vi "LookForStartOfMessage.vi"(8 "error in (no error)":errorcluster, 11 "TCP_Client in":refnum<class "TCP_Client.lvclass">) -> (0 "error out":errorcluster, 3 "TCP_Client out":refnum<class "TCP_Client.lvclass">)   [LabVIEW 2023, in "TCP_Client.lvlib" / "TCP_Client.lvclass"]
uses:
  TCP_Client.lvclass
  C:/Program Files (x86)/National Instruments/LabVIEW 2023/vi.lib/ActorFramework/Actor/Actor.lvclass
  <vilib>/ActorFramework/Actor/Actor.lvclass/Actor.ctl
  <vilib>/ActorFramework/Message Enqueuer/Message Enqueuer.lvclass/Message Enqueuer.ctl
  TCP_Client.lvclass/TCP_Client.ctl
  TCP_Client Messages/DisabelConnectButton Msg/DisabelConnectButton Msg.lvclass/DisabelConnectButton Msg.ctl
  <vilib>/ActorFramework/Message Enqueuer/Init from Existing Queue.vi
  <vilib>/ActorFramework/Message Enqueuer/Enqueue.vi
  TCP_Client Messages/LookForStartOfMessage Msg/LookForStartOfMessage Msg.lvclass
  C:/Program Files (x86)/National Instruments/LabVIEW 2023/vi.lib/ActorFramework/Message/Message.lvclass
  TCP_Client Messages/GetMessageLength Msg/GetMessageLength Msg.lvclass
  TCP_Client Messages/DisabelConnectButton Msg/DisabelConnectButton Msg.lvclass
  <vilib>/ActorFramework/Message Priority Queue/Priority Enqueue.vi
  <vilib>/ActorFramework/Message Enqueuer/Message Enqueuer.lvclass
  <vilib>/ActorFramework/Actor/Actor.lvclass
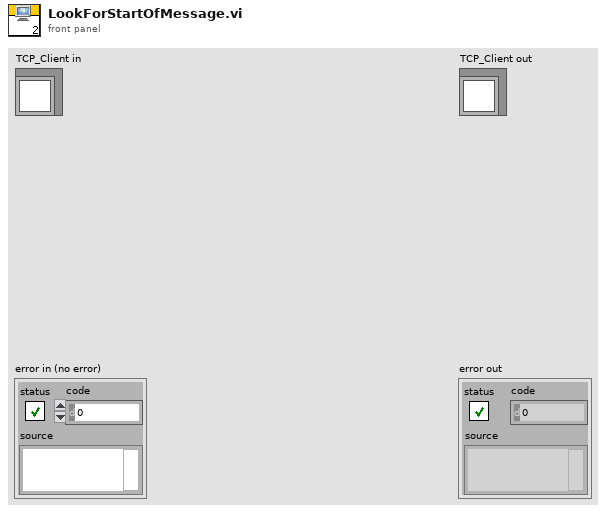
[diagram p1: front panel]
types:
  T1 = enum8{"Enabled", "Disabled", "Disabled and Grayed Out"}
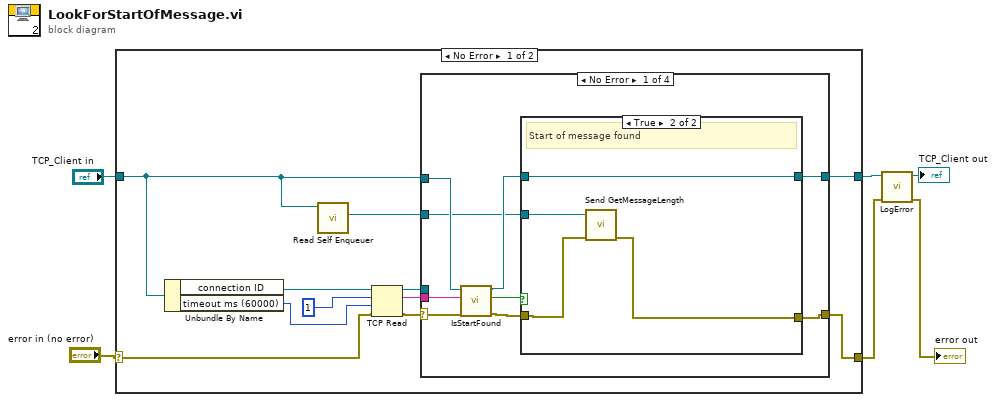
[diagram p0: block diagram]
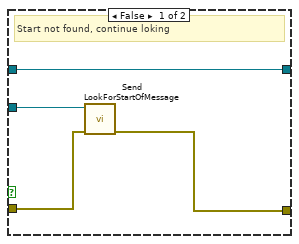
[diagram p2: hidden frame]
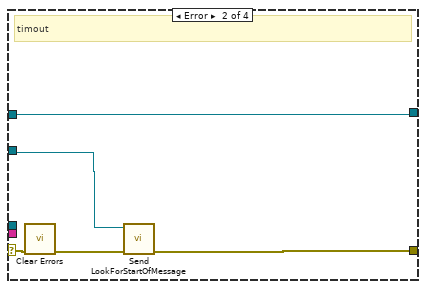
[diagram p3: hidden frame]
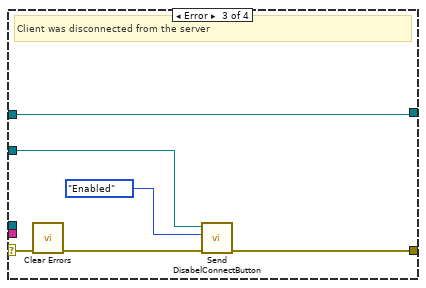
[diagram p4: hidden frame]
diagram:
  n1 = case shown="No Error" "error in (no error)" {
    selector: "error in (no error)" -> [w14 w49]
    tunnel: [w11 w49] -> w2
    tunnel: [w8 w48] -> w4
    tunnel: "TCP_Client in" -> [w9 w48]
    frame No Error {
      n2 = Unbundle By Name(w9) -> ("connection ID"=w17:refnum<k5>, "timeout ms (60000)"=w15:i32)
      n3 = call <vilib>:"Read Self Enqueuer.vi"("Actor"=w9) -> ("Self Enqueuer"=w10:refnum<class "Message Enqueuer.lvclass">)  [unwired: 10 in]
      n4 = TCP Read(connection ID=w17, bytes to read=1, error in (no error)=w14, 9:w15) -> (connection ID out=w13:refnum<k5>, data out=w12:string, error out=w7:errorcluster)  [unwired: 1 in]
      n5 = case shown="No Error" w7 {
        selector: w7 -> [w24 w39 w41 w46]
        tunnel: w13 -> [_ _ _ _]
        tunnel: w12 -> [w25 _ _ _]
        tunnel: [w20 w36 w42 w46] -> w11
        tunnel: w10 -> [w18 w35 w44 _]
        tunnel: w9 -> [w26 w38 w45 w47]
        tunnel: [w19 w38 w45 w47] -> w8
        frame No Error {
          n6 = call "IsStartFound.vi"("error in (no error)"=w24, "data in"=w25, "TCP_Client in"=w26) -> ("error out"=w21:errorcluster, "StartOfMessage"=w23:bool, "TCP_Client out"=w22:refnum<class "TCP_Client.lvclass">)  [unwired: 6 in]
          n7 = case shown="True" w23 {
            tunnel: w22 -> [w30 w34]
            tunnel: w21 -> [w28 w32]
            tunnel: [w27 w31] -> w20
            tunnel: [w30 w34] -> w19
            tunnel: w18 -> [w29 w33]
            frame False {
              # "Start not found, continue loking"
              n8 = call "Send LookForStartOfMessage.vi"("error in (no error)"=w28, "Message Enqueuer"=w29) -> ("error out"=w27:errorcluster)  [unwired: 8 in, 1 out]
            }
            frame True {
              # "Start of message found"
              n9 = call "Send GetMessageLength.vi"("error in (no error)"=w32, "Message Enqueuer"=w33) -> ("error out"=w31:errorcluster)  [unwired: 8 in, 1 out]
            }
          }
        }
        frame Error {
          # "timout"
          n10 = call <vilib>:"Clear Errors.vi"("error in (no error)"=w39) -> ("error out"=w37:errorcluster)  [unwired: 5 in, 1 out]
          n11 = call "Send LookForStartOfMessage.vi"("error in (no error)"=w37, "Message Enqueuer"=w35) -> ("error out"=w36:errorcluster)  [unwired: 8 in, 1 out]
        }
        frame Error {
          # "Client was disconnected from the server"
          n12 = call <vilib>:"Clear Errors.vi"("error in (no error)"=w41) -> ("error out"=w40:errorcluster)  [unwired: 5 in, 1 out]
          n13 = call "Send DisabelConnectButton.vi"("error in (no error)"=w40, "Connect button Disabled"=T1."Enabled", "Message Enqueuer"=w44) -> ("error out"=w42:errorcluster)  [unwired: 7 in, 1 out]
        }
        frame Default {
          # "Error will be sent to errorlog file"
        }
      }
    }
    frame Error {
    }
  }
  n14 = call "LogError.vi"("error in (no error)"=w2, "TCP_Client in"=w4) -> ("error out"=→"error out":errorcluster, "TCP_Client out"=→"TCP_Client out":refnum<class "TCP_Client.lvclass">)  [unwired: 8 in]
